vi "timestamp.vi"(0 "timestamp":dbl=1578559154.0 format="%#_14f", 2 "秒数的小数部分":dbl format="%#_13g") -> (7 "时间标识":timestamp)   [LabVIEW 2018]
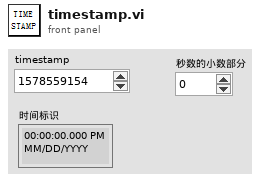
[diagram p1: front panel]
types:
  T1 = typedef "LVDateTimeRec.ctl" = cluster{"秒数的小数部分":dbl, "秒":i32, "分":i32, "时":i32, "日":i32, "月":i32, "年":i32, "天数（周）":i32, "天数（年）":i32, "DST":i32}
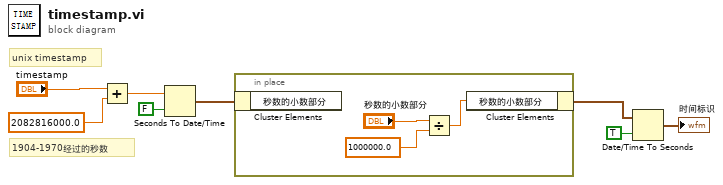
[diagram p0: block diagram]
diagram:
  # "unix timestamp"
  # "1904-1970经过的秒数"
  n1 = Add(x="timestamp", y=2082816000.0) -> (x+y=w7:dbl)
  n2 = Seconds To Date/Time(time stamp (now)=w7, to UTC (F)=FALSE ("转换为UTC (F)")) -> (date time rec=w2:T1)
  n3 = in-place {
    n4 = in-place-cluster #1(w2) -> ()  [unwired: 1 out]
    n5 = Divide(x="秒数的小数部分", y=1000000.0) -> (x/y=w9:dbl)
    n6 = in-place-cluster #1("秒数的小数部分"=w9) -> (w1:T1)
  }
  n7 = Date/Time To Seconds(1:TRUE ("是UTC (F)"), 2:w1) -> (0:→"时间标识":timestamp)
